vi "Lidar2XY (SubVI).vi"(6 "MaxRange":dbl=20000.0, 11 "Lidar":T1) -> (2 "Y":dbl[](array[numeric]), 3 "X":dbl[](array[numeric]))   [LabVIEW 2014]
types:
  T1 = cluster{"Magnitude":u16[], "Direction":fxp<+/-,16,8>[]}
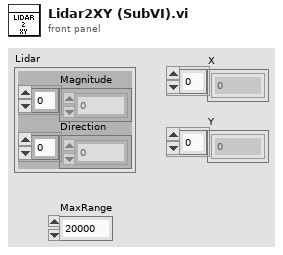
[diagram p1: front panel]
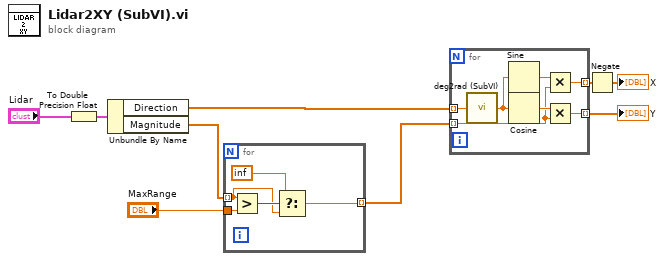
[diagram p0: block diagram]
diagram:
  n1 = To Double Precision Float(number="Lidar") -> (double precision float=w8:cluster{"Magnitude":dbl[], "Direction":dbl[]})
  n2 = Unbundle By Name(w8) -> ("Direction"=w9:dbl[], "Magnitude"=w2:dbl[])
  n3 = for {
    tunnel: w2 -> [w12] mode=indexing
    tunnel: "MaxRange" -> [w14]
    tunnel: [w10] -> w1 mode=indexing
    n4 = Greater?(x=w12, y=w14) -> (0:w13:bool)
    n5 = Select(t=inf, s=w13, f=w12) -> (s? t:f=w10:dbl)
  }
  n6 = for {
    tunnel: w9 -> [w17] mode=indexing
    tunnel: w1 -> [w15] mode=indexing
    tunnel: [w19] -> w6 mode=indexing
    tunnel: [w18] -> w7 mode=indexing
    n7 = call "deg2rad (SubVI).vi"("Angle [deg]"=w17) -> ("Angle[rad]"=w21:dbl)
    n8 = Sine(x=w21) -> (sin(x)=w16:dbl)
    n9 = Cosine(x=w21) -> (cos(x)=w20:dbl)
    n10 = Multiply(x=w16, y=w15) -> (x*y=w19:dbl)
    n11 = Multiply(x=w20, y=w15) -> (x*y=w18:dbl)
  }
  "Y" <- w7
  n12 = Negate(x=w6) -> (-x=→"X":dbl[])
